vi "STD.vi"(11 "Input_array":dbl[][](array[numeric])) -> (3 "STD":dbl[](array[numeric]))   [LabVIEW 2013]
uses:
  <vilib>/Analysis/NI_AALBase.lvlib
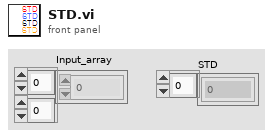
[diagram p1: front panel]
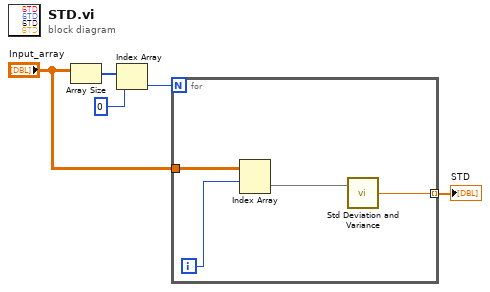
[diagram p0: block diagram]
diagram:
  n1 = Array Size(array="Input_array") -> (size(s)=w5:i32[])
  n2 = Index Array(array=w5, index=0) -> (element=w3:i32)
  n3 = for {
    N: w3 -> [_]
    tunnel: "Input_array" -> [w9]
    tunnel: [w6] -> w1 mode=indexing
    i -> [w8]
    n4 = Index Array(array=w9, index (row)=w8) -> (element=w7:dbl[])  [unwired: 1 in]
    n5 = call <vilib>:"Std Deviation and Variance.vi"("X"=w7) -> ("standard deviation"=w6:dbl)  [unwired: 1 in, 2 out]
  }
  "STD" <- w1
